vi "PCO_GetAcquireMode.vi"(8 "error in (no error)":errorcluster {"code" format="%x"}, 11 "ph":u64) -> (0 "error out":errorcluster {"code" format="%x"}, 1 "wAcquMode":u16(ring) items=["auto", "external", "external modulate"], 2 "ErrorMessage":i32 format="%x", 3 "ph out":u64)   [LabVIEW 2019, in "SDK.lvlib" / "RecordingControl.lvlib"]
doc: "<b>Description:</b>\nThis function returns the current acquire mode of the camera.\nAcquire mode can be either [auto], [external] or [external modulate].\n\n<b>Supported camera type:</b>\nAll cameras\n\n<b>Descriptor dependency:</b>\ndwGeneralCapsDESC1: NO_ACQUIREMODE"
uses:
  RecordingControl.lvlib
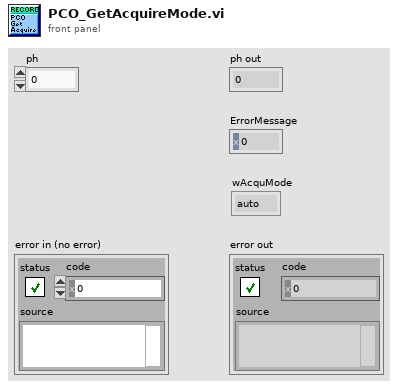
[diagram p1: front panel]
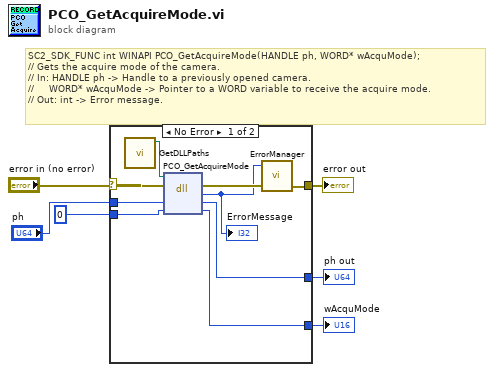
[diagram p0: block diagram]
diagram:
  # "SC2_SDK_FUNC int WINAPI PCO_GetAcquireMode(HANDLE ph, WORD* wAcquMode);\n// Gets the acquire mode of the camera.\n// In: HANDLE ph -> Handle to a previously opened camera.\n//     WORD* wAcquMode -> Pointer to a WORD variable to receive the acquire mode.\n// Out: int -> Error message."
  n1 = case shown="No Error" "error in (no error)" {
    selector: "error in (no error)" -> [w11 w16]
    tunnel: "ph" -> [w15 w18]
    tunnel: [w14 w18] -> w5
    tunnel: u16 0 ("wAcquMode") -> [w13 w17]
    tunnel: [w12 w17] -> w3
    tunnel: [w9 w16] -> w2
    frame No Error {
      n2 = call "GetDLLPaths.vi"() -> ("SC2_Cam_Path"=w7:path)  [unwired: 9 in, 2 out]
      n3 = dll-call lib="?" fn="PCO_GetAcquireMode"(path in=w7, error in=w11, "ph"=w15, "wAcquMode"=w13) -> (error out=w10:errorcluster, "return type"=w8:i32, "ph"=w14:u64, "wAcquMode"=w12:u16)  [unwired: 1 in, 1 out]
      "ErrorMessage" <- w8
      n4 = call "ErrorManager.vi"("error in (no error)"=w10, "error code"=w8) -> ("error out"=w9:errorcluster)  [unwired: 3 in]
    }
    frame Error {
    }
  }
  "ph out" <- w5
  "wAcquMode" <- w3
  "error out" <- w2
